vi "Cycle.vi"() -> ()   [LabVIEW 2020]
uses:
  Reset.ctl
  Cycle Status.ctl
  Grade Gate.ctl
  Traffic Signal.ctl
  PedX Signal.ctl
  Global Indicators.vi
panel:
  out "Cycle Status":T1
  in  "Reset":T2
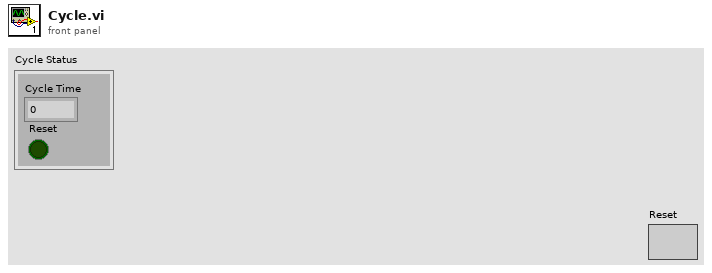
[diagram p1: front panel]
types:
  T1 = typedef "Cycle Status.ctl" = cluster{"Cycle Time":dbl, "Reset":bool}
  T2 = typedef "Reset.ctl" = bool
  T3 = typedef "PedX Signal.ctl" = cluster{"PedX Walk":bool, "PedX Stop":bool}
  T4 = typedef "Traffic Signal.ctl" = cluster{"Red Light":bool, "Yellow Light":bool, "Green Light":bool, "Yellow Turn":bool, "Green Turn":bool}
  T5 = enum16{"R-R", "NS Left G", "NS Left Y", "NS Straight G", "NS Straight Y"}
  T6 = typedef "Grade Gate.ctl" = cluster{"UP 2":bool, "Pivot":bool, "UP 3":bool, "UP 4":bool, "UP 5":bool, "UP 6":bool, "DOWN 2":bool, "DOWN 3":bool, "DOWN 4":bool, "DOWN 5":bool, "DOWN 6":bool, "DOWN 7":bool, "DOWN 8":bool, "SIDE 2":bool, "SIDE 3":bool, "SIDE 4":bool, "SIDE 5":bool, "Blinky 2":bool, "Blinky 1":bool}
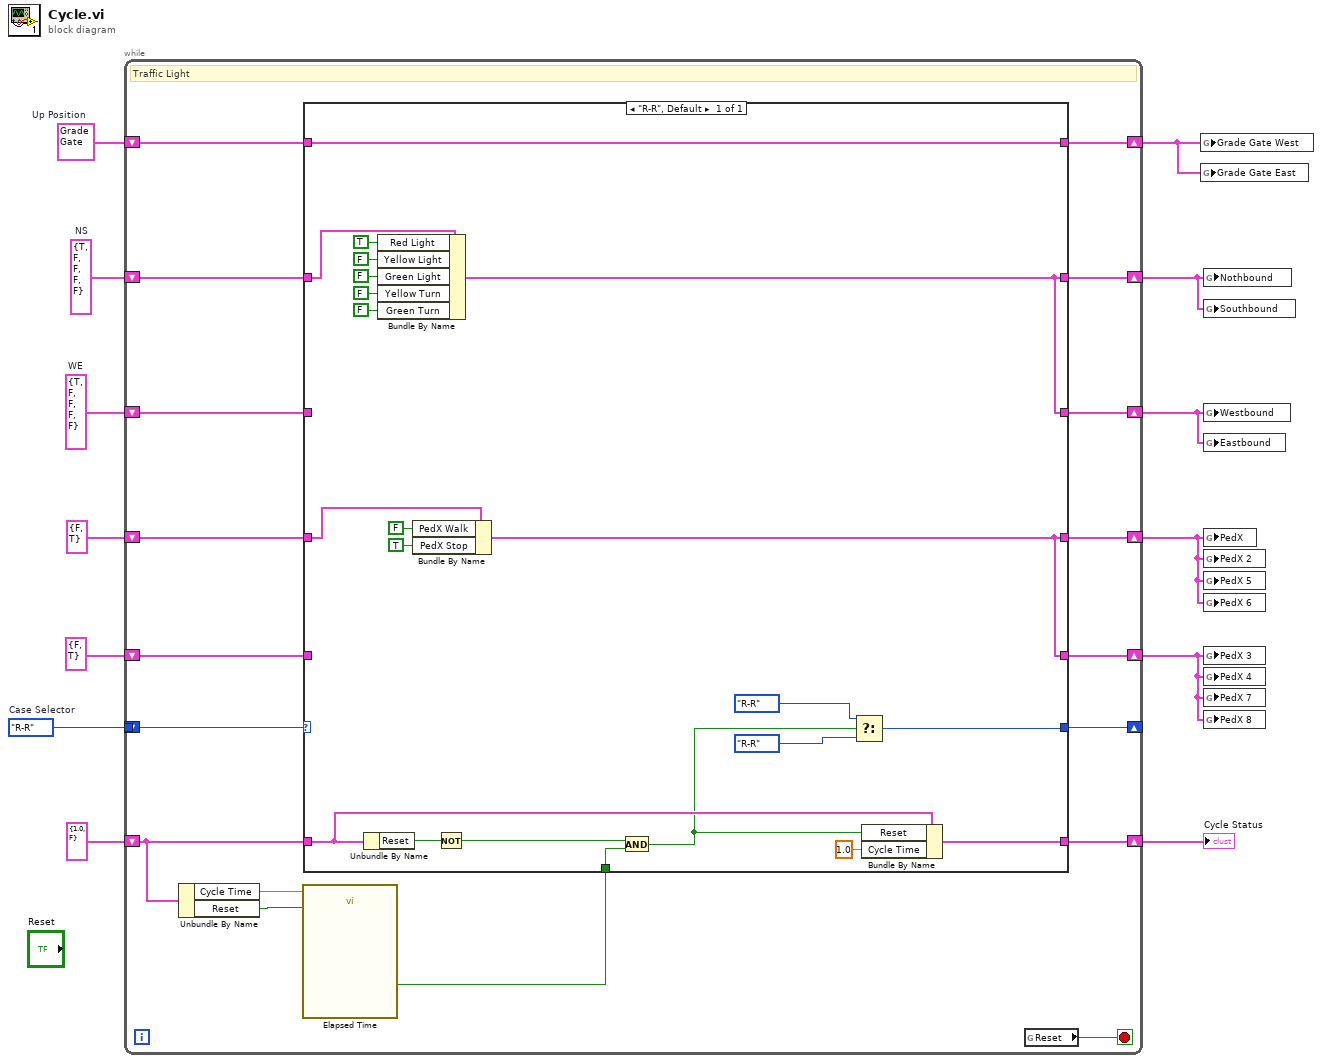
[diagram p0: block diagram]
diagram:
  w7 = T4 {"Red Light"=TRUE, "Yellow Light"=FALSE, "Green Light"=FALSE, "Yellow Turn"=FALSE, "Green Turn"=FALSE}  # WE
  w11 = T4 {"Red Light"=TRUE, "Yellow Light"=FALSE, "Green Light"=FALSE, "Yellow Turn"=FALSE, "Green Turn"=FALSE}  # NS
  w12 = T5."R-R"  # Case Selector
  w13 = T6 {"UP 2"=FALSE, "Pivot"=FALSE, "UP 3"=TRUE, "UP 4"=FALSE, "UP 5"=FALSE, "UP 6"=FALSE, "DOWN 2"=FALSE, "DOWN 3"=FALSE, "DOWN 4"=FALSE, "DOWN 5"=FALSE, "DOWN 6"=FALSE, "DOWN 7"=FALSE, "DOWN 8"=FALSE, "SIDE 2"=FALSE, "SIDE 3"=FALSE, "SIDE 4"=FALSE, "SIDE 5"=FALSE, "Blinky 2"=FALSE, "Blinky 1"=FALSE}  # Up Position
  n1 = while {
    shift-right: [w31] -> w10
    shift-left: w13 -> [w30]
    tunnel: w12 -> [w29]
    shift-right: [w28] -> w9
    shift-left: w11 -> [w27]
    shift-right: [w26] -> w8
    shift-left: w7 -> [w25]
    shift-right: [w24] -> w5
    shift-left: T3 {"PedX Walk"=FALSE, "PedX Stop"=TRUE} ("PedX") -> [w23]
    shift-right: [w21] -> w3
    shift-left: T3 {"PedX Walk"=FALSE, "PedX Stop"=TRUE} ("PedX") -> [w22]
    shift-right: [w20] -> w2
    shift-left: T1 {"Cycle Time"=1.0, "Reset"=FALSE} ("Cycle Status") -> [w17]
    shift-right: [w16] -> _
    shift-left: _ -> [_]
    stop <- w14 stop-if-true
    # "Traffic Light"
    n2 = Unbundle By Name(w17) -> ("Cycle Time"=w19:dbl, "Reset"=w18:bool)
    n3 = call "Elapsed Time"("Time Target (s)"=w19, "Reset"=w18) -> ("Time has Elapsed"=w15:bool)  [unwired: 10 in, 7 out]
    n4 = case shown="\"R-R\", Default" w29 {
      tunnel: [w53] -> w31
      tunnel: w30 -> [w53]
      tunnel: [w46] -> w28
      tunnel: w27 -> [w52]
      tunnel: [w46] -> w26
      tunnel: w25 -> [_]
      tunnel: [w42] -> w24
      tunnel: w23 -> [w45]
      tunnel: w22 -> [_]
      tunnel: [w42] -> w21
      tunnel: [w35] -> w20
      tunnel: w17 -> [w34]
      tunnel: [w38] -> w16
      tunnel: w15 -> [w39]
      frame "R-R", Default {
        n5 = Unbundle By Name(w34) -> ("Reset"=w41:bool)
        n6 = Bundle By Name(cluster=w52, "Red Light"=TRUE, "Yellow Light"=FALSE, "Green Light"=FALSE, "Yellow Turn"=FALSE, "Green Turn"=FALSE) -> (w46:T4)
        n7 = Bundle By Name(cluster=w45, "PedX Walk"=FALSE, "PedX Stop"=TRUE) -> (w42:T3)
        n8 = Not(x=w41) -> (.not. x?=w40:bool)
        n9 = And(x=w40, y=w39) -> (x .and. y?=w33:bool)
        n10 = Select(t=T5."R-R" ("Case Selector"), s=w33, f=T5."R-R" ("Case Selector")) -> (s? t:f=w38:T5)
        n11 = Bundle By Name(cluster=w34, "Reset"=w33, "Cycle Time"=1.0) -> (w35:T1)
      }
    }
    n12 = global read "Global Indicators.vi" "Reset"() -> (w14:T2)
  }
  "Cycle Status" <- w2
  n13 = global write "Global Indicators.vi" "Grade Gate West"(w10) -> ()
  n14 = global write "Global Indicators.vi" "Grade Gate East"(w10) -> ()
  n15 = global write "Global Indicators.vi" "Nothbound"(w9) -> ()
  n16 = global write "Global Indicators.vi" "Southbound"(w9) -> ()
  n17 = global write "Global Indicators.vi" "Westbound"(w8) -> ()
  n18 = global write "Global Indicators.vi" "Eastbound"(w8) -> ()
  n19 = global write "Global Indicators.vi" "PedX"(w5) -> ()
  n20 = global write "Global Indicators.vi" "PedX 2"(w5) -> ()
  n21 = global write "Global Indicators.vi" "PedX 5"(w5) -> ()
  n22 = global write "Global Indicators.vi" "PedX 6"(w5) -> ()
  n23 = global write "Global Indicators.vi" "PedX 3"(w3) -> ()
  n24 = global write "Global Indicators.vi" "PedX 4"(w3) -> ()
  n25 = global write "Global Indicators.vi" "PedX 7"(w3) -> ()
  n26 = global write "Global Indicators.vi" "PedX 8"(w3) -> ()
